vi "Tosca-Start.vi"(11 "error in (no error)":errorcluster) -> (15 "error out":errorcluster)   [LabVIEW 2020]
uses:
  epl-vi-lib/PXI DAQ VIs/AODO/Typedefs/AODO-Action.ctl
  PXI DAQ VIs/TDT VIs/TDT AODO VIs/Typedefs/TDT-AODO-Action.ctl
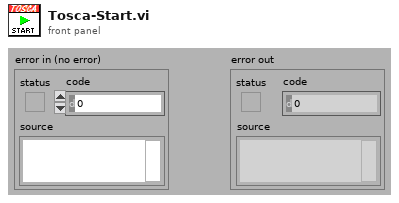
[diagram p1: front panel]
types:
  T1 = typedef "TDT-AODO-Action.ctl" = enum16{"Configure", "Initialize", "Start", "Stop", "Write", "Clean up", "Space available"}
  T2 = typedef "AODO-Action.ctl" = enum16{"Configure", "Initialize", "Start", "Write", "Clean up", "Init & Start", "Config & Test", "Position", "Set AO Gains", "Zero"}
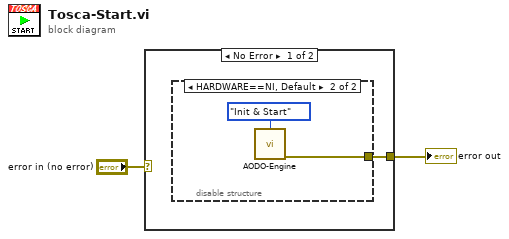
[diagram p0: block diagram]
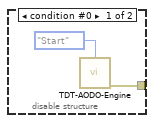
[diagram p2: hidden frame]
diagram:
  n1 = case shown="No Error" "error in (no error)" {
    selector: "error in (no error)" -> [_ w8]
    tunnel: [w3 w8] -> w1
    frame No Error {
      n2 = disable-structure shown="HARDWARE==NI, Default" {
        disable-tunnel: [w5 w6] -> w3
        frame condition #0 {
          n3 = call "TDT-AODO-Engine.vi"("Action"=TDT-AODO-Action."Start") -> ("error out"=w5:errorcluster)  [unwired: 12 in, 2 out]
        }
        frame condition #1 (active) {
          n4 = call "AODO-Engine.vi"("Action"=AODO-Action."Init & Start") -> ("error out"=w6:errorcluster)  [unwired: 12 in, 2 out]
        }
      }
    }
    frame Error {
    }
  }
  "error out" <- w1
